vi "Data for Dashboard.vi"() -> ()   [LabVIEW 2013]
panel:
  in  "Angle":dbl
  in  "Shot Count":dbl
  in  "Loaded":bool
  in  "Winch Power":bool
  in  "Winch Armed?":bool
  in  "Roller Direction":bool
  in  "Rollers on?":bool
  in  "Gyro?":bool
  in  "Flip Axes?":bool
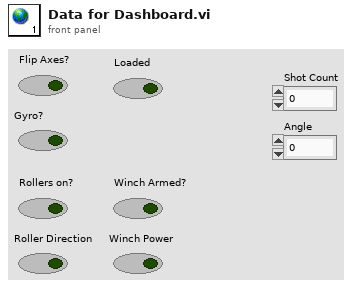
[diagram p1: front panel]
diagram:
